vi "PH_BeamlineController.get Target Attributes.vi"(0 "VI in":refnum<vi>, 2 "Target":T1, 5 "error in (no error)":errorcluster) -> (14 "VI out":refnum<vi>, 17 "Target Index":i32, 18 "Target Attributes":T2, 19 "error out":errorcluster)   [LabVIEW 2014, in "PH_BeamlineController.lvlib"]
uses:
  PH_BeamlineController.lvlib
  PH_BeamlineController.Target Attributes.ctl
  PH_BeamlineController.Targets.ctl
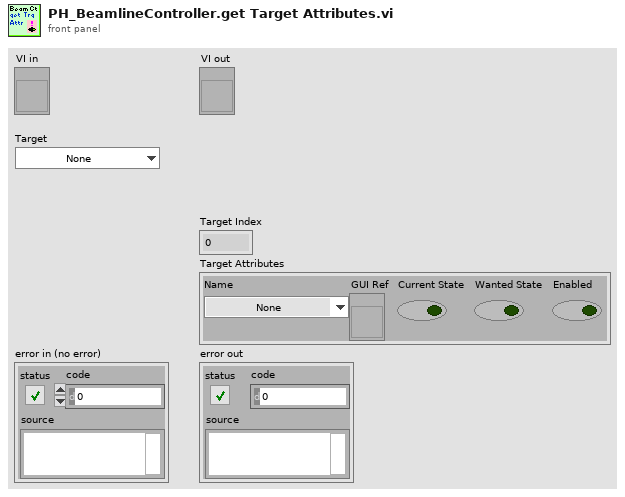
[diagram p1: front panel]
types:
  T1 = typedef "PH_BeamlineController.lvlib/PH_BeamlineController.Targets.ctl" = enum16{"None", "PreAmp", "Dump Exp Laserlab", "Exp Laserlab", "Calorimeter", "Dump Exp Laserbay", "Exp Laserbay", "Dump Exp Z6", "Exp Z6"}
  T2 = typedef "PH_BeamlineController.lvlib/PH_BeamlineController.Target Attributes.ctl" = cluster{"Name":T1, "GUI Ref":refnum<vi>, "Current State":bool, "Wanted State":bool, "Enabled":bool}
  T3 = typedef "PH_BeamlineController.lvlib/PH_BeamlineController.i attribute.ctl" = cluster{"Vacuum Exp LB":cluster{"Channel":string, "Limit [mbar]":dbl, "Pressure [mbar]":dbl, "GUI Ref":refnum<vi>}, "Sources":T4[], "PA DP Targets":T6[], "Path":cluster{"Source":T5, "PA DP Target":T7, "Target":T1}, "Targets":cluster{"Name":T1, "GUI Ref":refnum<vi>, "Current State":bool, "Wanted State":bool, "Enabled":bool}[], "Status Tags":cluster{"Name":string, "Status":T8}[], "special GUI Refs":T9}
  T4 = typedef "PH_BeamlineController.lvlib/PH_BeamlineController.Source Attributes.ctl" = cluster{"Name":T5, "GUI Ref":refnum<vi>, "Current State":bool, "Wanted State":bool}
  T5 = typedef "PH_BeamlineController.lvlib/PH_BeamlineController.Sources.ctl" = enum16{"None", "YLF", "fs-Frontend", "ns-Frontend", "YLF and ns-Frontend", "fs- and ns-Frontend"}
  T6 = typedef "PH_BeamlineController.lvlib/PH_BeamlineController.PA DP Target Attributes.ctl" = cluster{"Name":T7, "GUI Ref":refnum<vi>, "Current State":bool, "Wanted State":bool, "Enabled":bool}
  T7 = typedef "PH_BeamlineController.lvlib/PH_BeamlineController.PA DP Targets.ctl" = enum16{"None", "Dump PA Delayed Beam", "Dump PA Undelayed Beam", "Dumps PA Delayed and Undelayed Beam"}
  T8 = typedef "PH_StatusHandler.lvlib/PH_StatusHandler.Status.ctl" = i16
  T9 = typedef "PH_BeamlineController.lvlib/PH_BeamlineController.special GUI Refs.ctl" = cluster{"PA-Backreflection-Meas":refnum<vi>, "fs_Synchrolock_Watch":refnum<vi>}
  T10 = cluster{"Name":T1, "GUI Ref":refnum<vi>, "Current State":bool, "Wanted State":bool, "Enabled":bool}[]
  T11 = cluster{"Name":T1, "GUI Ref":refnum<vi>, "Current State":bool, "Wanted State":bool, "Enabled":bool}
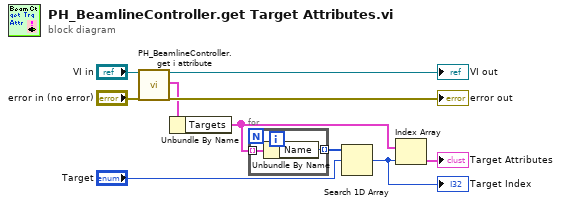
[diagram p0: block diagram]
diagram:
  n1 = call "PH_BeamlineController.get i attribute.vi"("i ref in"="VI in", "error in (no error)"="error in (no error)") -> ("i ref out"=→"VI out":refnum<vi>, "i attribute"=w4:T3, "error out"=→"error out":errorcluster)  [unwired: 15 in]
  n2 = Unbundle By Name(w4) -> ("Targets"=w2:T10)
  n3 = for {
    tunnel: w2 -> [w12] mode=indexing
    tunnel: [w11] -> w1 mode=indexing
    n4 = Unbundle By Name(w12) -> ("Name"=w11:T1)
  }
  n5 = Search 1D Array(1D array=w1, element="Target") -> (index of element=w3:i32)  [unwired: 1 in]
  "Target Index" <- w3
  n6 = Index Array(array=w2, index=w3) -> (element=→"Target Attributes":T11)
